vi "Window Hanning.vi"(1 "Normalize? (False)":bool, 2 "N":i32) -> (0 "window":dbl[](array[numeric]))   [LabVIEW 2020, in "FFTWDLL.lvlib"]
doc: "Hanning function (coherent mode - period N samples)."
uses:
  FFTWDLL.lvlib
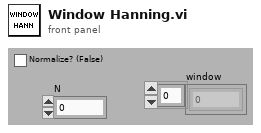
[diagram p1: front panel]
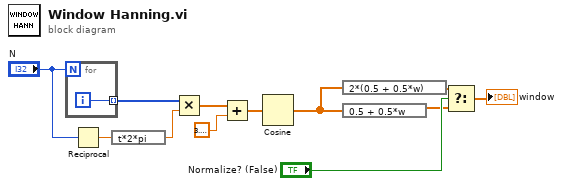
[diagram p0: block diagram]
diagram:
  n1 = for {
    N: "N" -> [_]
    tunnel: [w13] -> w10 mode=indexing
    i -> [w13]
  }
  n2 = Reciprocal(x="N") -> (1/x=w11:dbl)
  n3 = expression code="t*2*pi"(w11) -> (w9:dbl)
  n4 = Multiply(x=w10, y=w9) -> (x*y=w8:dbl[])
  n5 = Add(x=w8, y=3.141592653589793) -> (x+y=w6:dbl[])
  n6 = Cosine(x=w6) -> (cos(x)=w1:dbl[])
  n7 = expression code="2*(0.5 + 0.5*w)"(w1) -> (w4:dbl[])
  n8 = expression code="0.5 + 0.5*w"(w1) -> (w3:dbl[])
  n9 = Select(t=w4, s="Normalize? (False)", f=w3) -> (s? t:f=→"window":dbl[])
